vi "ShutDown.vi"(8 "error in":errorcluster, 11 "Super Data Model":refnum<class "Super Data Model.lvclass">) -> (0 "error out":errorcluster)   [LabVIEW 2013, in "Modbus Library - Advance.lvlib" / "Super Data Model.lvclass"]
uses:
  Super Data Model.lvclass
  Standard Data Model/Standard Data Model.lvclass
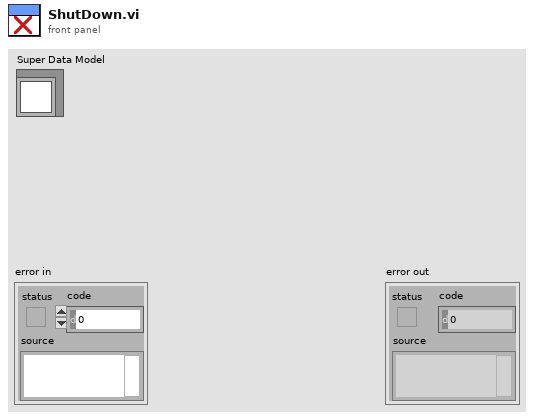
[diagram p1: front panel]
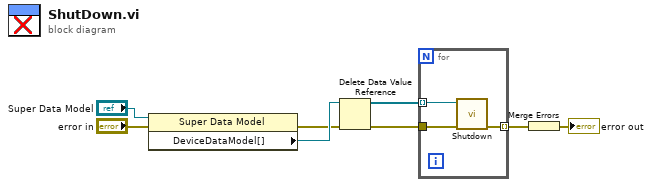
[diagram p0: block diagram]
diagram:
  n1 = property class="Super Data Model"(reference="Super Data Model", error in="error in") -> (error out=w1:errorcluster, "DeviceDataModel[]"=w6:refnum<data-value>)  [unwired: 1 out]
  n2 = Delete Data Value Reference(data value reference=w6, error in=w1) -> (data value=w5:refnum<class "Standard Data Model.lvclass">[], error out=w4:errorcluster)
  n3 = for {
    tunnel: w4 -> [w11]
    tunnel: [w10] -> w8 mode=indexing
    tunnel: w5 -> [w9] mode=indexing
    n4 = call-dynamic "Shutdown.vi"("error in"=w11, "device data model in"=w9) -> ("error out"=w10:errorcluster)  [unwired: 9 in]
  }
  n5 = Merge Errors(w8) -> (→"error out":errorcluster)
